vi "Global Variables Clear.vi"   [LabVIEW 2018]
uses:
  Global Variables.vi
panel:
  # "CLEAR GLOBAL DATA"
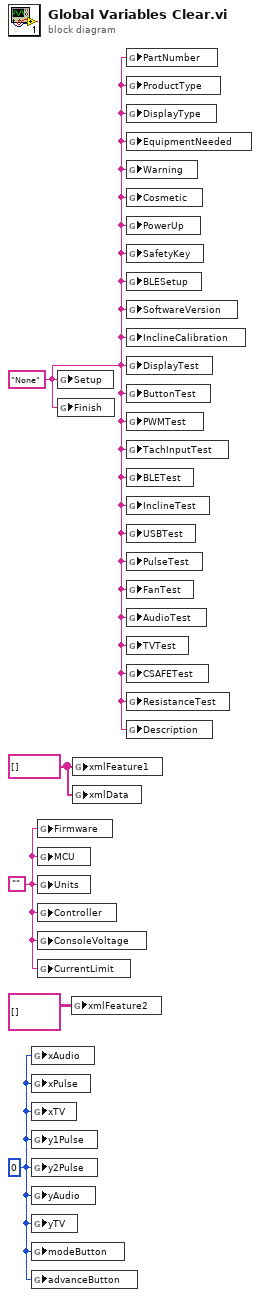
[diagram p0: block diagram]
diagram:
  w2 = "None"
  w3 = ""
  w1 = 0
  w4 = string[] []
  n1 = global write "Global Variables.vi" "xAudio"(w1) -> ()
  n2 = global write "Global Variables.vi" "xPulse"(w1) -> ()
  n3 = global write "Global Variables.vi" "xTV"(w1) -> ()
  n4 = global write "Global Variables.vi" "y1Pulse"(w1) -> ()
  n5 = global write "Global Variables.vi" "y2Pulse"(w1) -> ()
  n6 = global write "Global Variables.vi" "yAudio"(w1) -> ()
  n7 = global write "Global Variables.vi" "yTV"(w1) -> ()
  n8 = global write "Global Variables.vi" "modeButton"(w1) -> ()
  n9 = global write "Global Variables.vi" "advanceButton"(w1) -> ()
  n10 = global write "Global Variables.vi" "Firmware"(w3) -> ()
  n11 = global write "Global Variables.vi" "MCU"(w3) -> ()
  n12 = global write "Global Variables.vi" "Units"(w3) -> ()
  n13 = global write "Global Variables.vi" "Controller"(w3) -> ()
  n14 = global write "Global Variables.vi" "ConsoleVoltage"(w3) -> ()
  n15 = global write "Global Variables.vi" "CurrentLimit"(w3) -> ()
  n16 = global write "Global Variables.vi" "Setup"(w2) -> ()
  n17 = global write "Global Variables.vi" "Finish"(w2) -> ()
  n18 = global write "Global Variables.vi" "xmlFeature2"(string[][] []) -> ()
  n19 = global write "Global Variables.vi" "xmlFeature1"(w4) -> ()
  n20 = global write "Global Variables.vi" "xmlData"(w4) -> ()
  n21 = global write "Global Variables.vi" "PartNumber"(w2) -> ()
  n22 = global write "Global Variables.vi" "ProductType"(w2) -> ()
  n23 = global write "Global Variables.vi" "DisplayType"(w2) -> ()
  n24 = global write "Global Variables.vi" "EquipmentNeeded"(w2) -> ()
  n25 = global write "Global Variables.vi" "Warning"(w2) -> ()
  n26 = global write "Global Variables.vi" "Cosmetic"(w2) -> ()
  n27 = global write "Global Variables.vi" "PowerUp"(w2) -> ()
  n28 = global write "Global Variables.vi" "SafetyKey"(w2) -> ()
  n29 = global write "Global Variables.vi" "BLESetup"(w2) -> ()
  n30 = global write "Global Variables.vi" "SoftwareVersion"(w2) -> ()
  n31 = global write "Global Variables.vi" "InclineCalibration"(w2) -> ()
  n32 = global write "Global Variables.vi" "DisplayTest"(w2) -> ()
  n33 = global write "Global Variables.vi" "ButtonTest"(w2) -> ()
  n34 = global write "Global Variables.vi" "PWMTest"(w2) -> ()
  n35 = global write "Global Variables.vi" "TachInputTest"(w2) -> ()
  n36 = global write "Global Variables.vi" "BLETest"(w2) -> ()
  n37 = global write "Global Variables.vi" "InclineTest"(w2) -> ()
  n38 = global write "Global Variables.vi" "USBTest"(w2) -> ()
  n39 = global write "Global Variables.vi" "PulseTest"(w2) -> ()
  n40 = global write "Global Variables.vi" "FanTest"(w2) -> ()
  n41 = global write "Global Variables.vi" "AudioTest"(w2) -> ()
  n42 = global write "Global Variables.vi" "TVTest"(w2) -> ()
  n43 = global write "Global Variables.vi" "CSAFETest"(w2) -> ()
  n44 = global write "Global Variables.vi" "ResistanceTest"(w2) -> ()
  n45 = global write "Global Variables.vi" "Description"(w2) -> ()
